vi "根据一字槽的缺口计算旋转矩形找边-计算一字槽角度.vi"(9 "存储缺口位置 out":cluster{"X":sgl, "Y":sgl}[](array[cluster]), 11 "Img输入":T1) -> (0 "一字槽角度线":T2, 1 "角度差异":dbl[](array[numeric]), 2 "一字槽角度":dbl, 3 "Img out":T1, 4 "一字槽宽度":dbl)   [LabVIEW 2014]
uses:
  <vilib>/vision/Measure.llb/Edge Options.ctl
  <vilib>/vision/Measure.llb/Edge Polarity.ctl
  <vilib>/vision/Image Controls.llb/IMAQ Image.ctl
  <vilib>/vision/NI_Vision_Development_Module.lvlib
panel:
  out "Angle2":dbl
  out "Angle1":dbl
  out "角度 2":dbl
  out "角度":dbl
  out "缺口连线角度":dbl
  out "?":dbl[](array[numeric])
  out "槽边与缺口连线差异":dbl
  out "两槽边角度差异":dbl
  in  "Options2":T5={"Search Direction"=1, "Edge Options"={"Edge Polarity"=1, "Kernel Size"=9, "Width"=5, "Minimum Edge Strength"=15.0, "Interpolation Type"=enum."Bilinear Fixed", "Data Processing Method"=enum."Average"}, "Show Search Area"=TRUE, "Show Search Lines"=FALSE, "Show Edges Found"=FALSE, "Show Result"=TRUE, "Search Area Color"=65280, "Search Lines Color"=255, "Edge Locations Color"=16776960, "Result Color"=16711680, "Overlay Group Name"=""} {"Edge Options"."Edge Polarity" items=["All Edges", "Rising Edges", "Falling Edges"]; "Edge Options"."Minimum Edge Strength" format="%.2f"; "Edge Options"."Width" step=2; "Edge Options"."Kernel Size" step=2; "Search Direction" items=["Left to Right", "Right to Left", "Top to Bottom", "Bottom to Top"]}
  in  "Options输入":T5={"Search Direction"=0, "Edge Options"={"Edge Polarity"=1, "Kernel Size"=9, "Width"=3, "Minimum Edge Strength"=15.0, "Interpolation Type"=enum."Bilinear Fixed", "Data Processing Method"=enum."Average"}, "Show Search Area"=TRUE, "Show Search Lines"=FALSE, "Show Edges Found"=FALSE, "Show Result"=TRUE, "Search Area Color"=65280, "Search Lines Color"=255, "Edge Locations Color"=16776960, "Result Color"=16711680, "Overlay Group Name"=""} {"Edge Options"."Edge Polarity" items=["All Edges", "Rising Edges", "Falling Edges"]; "Edge Options"."Minimum Edge Strength" format="%.2f"; "Edge Options"."Width" step=2; "Edge Options"."Kernel Size" step=2; "Search Direction" items=["Left to Right", "Right to Left", "Top to Bottom", "Bottom to Top"]}
  out "两缺口连线角度":dbl
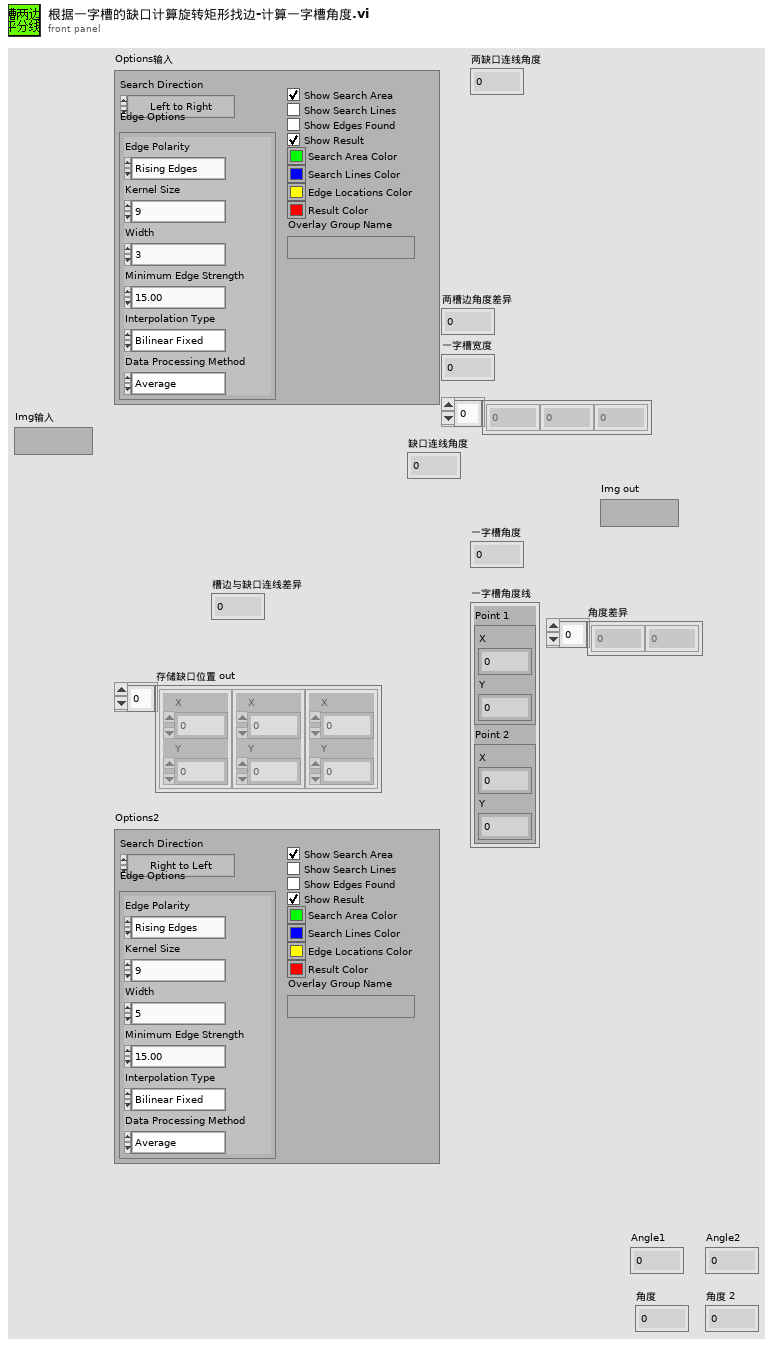
[diagram p1: front panel]
types:
  T1 = typedef "IMAQ Image.ctl" = refnum<image>
  T2 = cluster{"Point 1":cluster{"X":sgl, "Y":sgl}, "Point 2":cluster{"X":sgl, "Y":sgl}}
  T3 = typedef "Edge Options.ctl" = cluster{"Edge Polarity":T4, "Kernel Size":u32, "Width":u32, "Minimum Edge Strength":sgl, "Interpolation Type":enum32{"Zero Order", "Bilinear", "Quadratic", "Cubic", "Bilinear Fixed"}, "Data Processing Method":enum32{"Average", "Median"}}
  T4 = typedef "Edge Polarity.ctl" = u32
  T5 = cluster{"Search Direction":u32, "Edge Options":T3, "Show Search Area":bool, "Show Search Lines":bool, "Show Edges Found":bool, "Show Result":bool, "Search Area Color":u32, "Search Lines Color":u32, "Edge Locations Color":u32, "Result Color":u32, "Overlay Group Name":string}
  T6 = cluster{"Center (Pixels)":cluster{"X":sgl, "Y":sgl}, "Center (Pixels)":cluster{"X":sgl, "Y":sgl}}
  T7 = typedef "ROI Descriptor" = cluster{"Global Rectangle":i32[], "Contours":cluster{"ID":enum32{"External", "Internal"}, "Type":u32, "Coordinates":i32[]}[]}
  T8 = cluster{"Point1 (Pixels)":cluster{"X":sgl, "Y":sgl}, "Point2 (Pixels)":cluster{"X":sgl, "Y":sgl}, "Point1 (Real-World)":cluster{"X":sgl, "Y":sgl}, "Point2 (Real-World)":cluster{"X":sgl, "Y":sgl}, "Angle (Pixel)":dbl, "Angle (Real-World)":dbl, "Score":dbl, "Straightness":dbl, "Average SNR (db)":dbl, "Calibration Valid":bool}[]
  T9 = cluster{"Point1 (Pixels)":cluster{"X":sgl, "Y":sgl}, "Point2 (Pixels)":cluster{"X":sgl, "Y":sgl}, "Point1 (Real-World)":cluster{"X":sgl, "Y":sgl}, "Point2 (Real-World)":cluster{"X":sgl, "Y":sgl}, "Angle (Pixel)":dbl, "Angle (Real-World)":dbl, "Score":dbl, "Straightness":dbl, "Average SNR (db)":dbl, "Calibration Valid":bool}
  T10 = cluster{"Point1 (Pixels)":cluster{"X":sgl, "Y":sgl}, "Point2 (Pixels)":cluster{"X":sgl, "Y":sgl}}
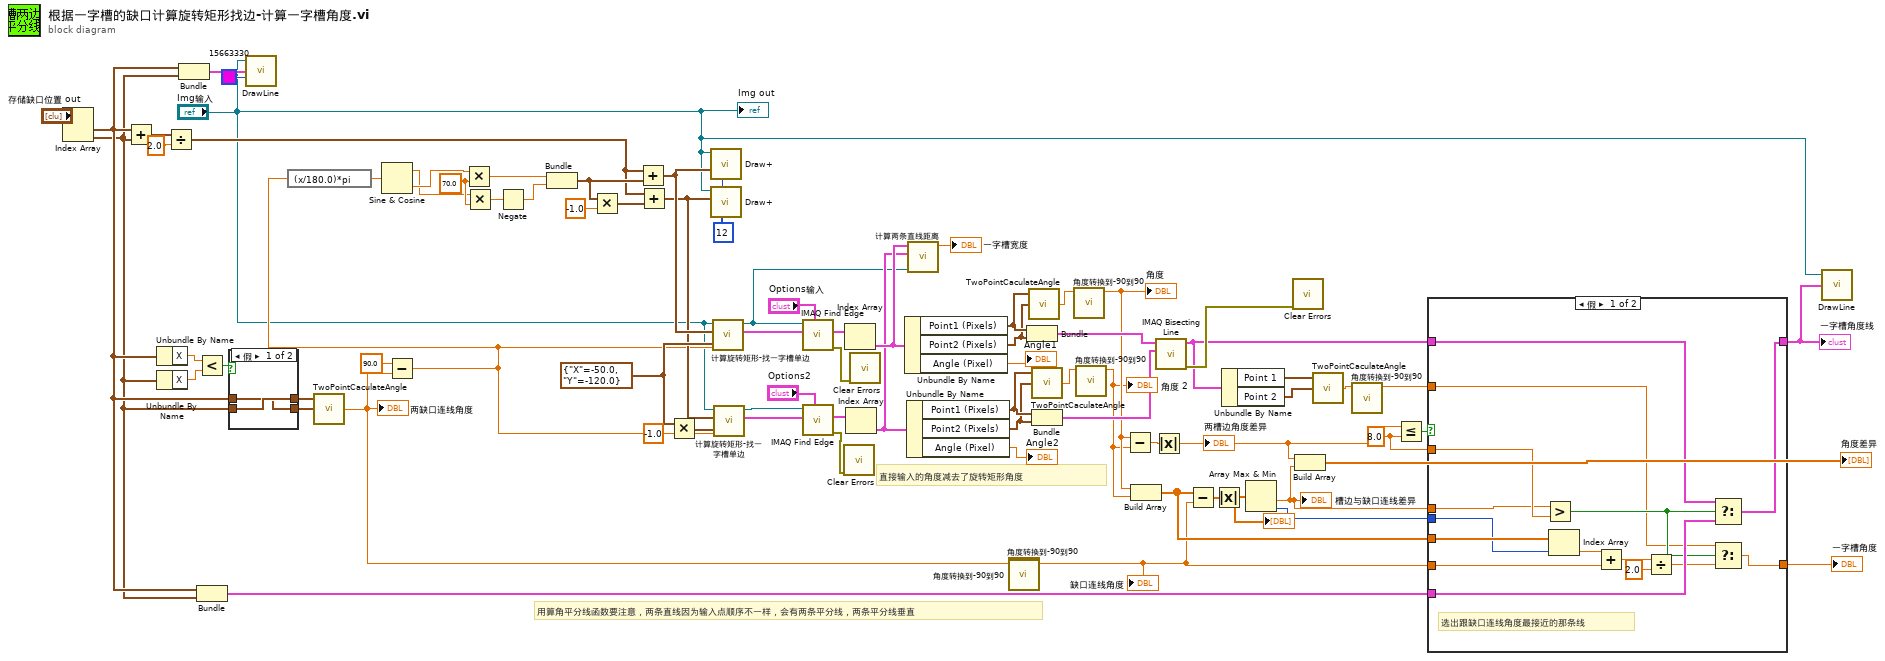
[diagram p0: block diagram]
diagram:
  w29 = 8.0 ("y")
  w45 = 12 ("Width")
  w56 = 70.0 ("y")
  w43 = cluster{"X":dbl, "Y":dbl} {"X"=-50.0, "Y"=-120.0} ("y")
  # "直接输入的角度减去了旋转矩形角度"
  # "用算角平分线函数要注意，两条直线因为输入点顺序不一样，会有两条平分线，两条平分线垂直"
  n1 = Index Array(array="存储缺口位置 out") -> (element #1=w20:cluster{"X":sgl, "Y":sgl}, element #2=w19:cluster{"X":sgl, "Y":sgl})  [unwired: 2 in]
  n2 = Add(x=w20, y=w19) -> (x+y=w63:cluster{"X":sgl, "Y":sgl})
  n3 = Unbundle By Name(w20) -> ("X"=w65:sgl)
  n4 = Unbundle By Name(w19) -> ("X"=w66:sgl)
  n5 = Divide(x=w63, y=2.0) -> (x/y=w50:cluster{"X":dbl, "Y":dbl})
  n6 = Bundle("Center (Pixels)"=w20, "Center (Pixels)"=w19) -> (w49:T6)  [unwired: 1 in]
  n7 = Less?(x=w65, y=w66) -> (x < y?=w67:bool)
  n8 = Bundle("Center (Pixels)"=w20, "Center (Pixels)"=w19) -> (w18:T6)  [unwired: 1 in]
  n9 = case shown="假" w67 {
    tunnel: w20 -> [w79 w82]
    tunnel: w19 -> [w80 w81]
    tunnel: [w80 w82] -> w68
    tunnel: [w79 w81] -> w69
    frame False {
    }
    frame True {
    }
  }
  n10 = call "DrawLine.vi"("Color"=u32 15663330, "Edge Points"=w49, "img in"="Img输入") -> ()  [unwired: 1 out]
  n11 = call "TwoPointCaculateAngle.vi"("Point2"=w69, "Point1"=w68) -> ("角度"=w11:dbl)  [unwired: 1 in]
  "两缺口连线角度" <- w11
  n12 = Subtract(x=90.0, y=w11) -> (x-y=w38:dbl)
  n13 = expression code="(x/180.0)*pi" ("degrees to radians")(w38) -> (w42:dbl)
  n14 = Sine & Cosine(0:w42) -> (1:w47:dbl, 2:w48:dbl)
  n15 = Multiply(x=w48, y=w56) -> (x*y=w57:dbl)
  n16 = Multiply(x=w47, y=w56) -> (x*y=w55:dbl)
  n17 = Negate(x=w55) -> (-x=w54:dbl)
  n18 = Bundle(w57, w54) -> (w53:cluster{dbl, dbl})  [unwired: 1 in]
  n19 = Multiply(x=w53, y=-1.0) -> (x*y=w51:cluster{dbl, dbl})
  n20 = Add(x=w50, y=w53) -> (x+y=w46:cluster{dbl, dbl})
  n21 = Add(x=w50, y=w51) -> (x+y=w39:cluster{dbl, dbl})
  n22 = Multiply(x=w43, y=-1.0) -> (x*y=w40:cluster{"X":dbl, "Y":dbl})
  n23 = call "Draw+.vi"("Width"=w45, "input cluster"=w46, "Image In"="Img输入") -> ()  [unwired: 3 in, 1 out]
  n24 = call "Draw+.vi"("Width"=w45, "input cluster"=w39, "Image In"="Img输入") -> ()  [unwired: 3 in, 1 out]
  n25 = call "计算旋转矩形-找一字槽单边.vi"("矩形"=w43, "旋转角度"=w38, "矩形中心"=w46, "Img输入"="Img输入") -> ("ROI Descriptor"=w37:T7, "Image Out"=w12:T1)  [unwired: 6 in]
  n26 = call "计算旋转矩形-找一字槽单边.vi"("矩形"=w40, "旋转角度"=w38, "矩形中心"=w39, "Img输入"="Img输入") -> ("ROI Descriptor"=w36:T7, "Image Out"=w35:T1)  [unwired: 6 in]
  n27 = call "IMAQ Find Edge"("Options"="Options输入", "ROI Descriptor"=w37, "Image"=w12) -> ("error out"=w17:errorcluster, "Straight Edges"=w72:T8)  [unwired: 5 in, 2 out]
  n28 = call "IMAQ Find Edge"("Options"="Options2", "ROI Descriptor"=w36, "Image"=w35) -> ("error out"=w16:errorcluster, "Straight Edges"=w73:T8)  [unwired: 5 in, 2 out]
  n29 = call <vilib>:"Clear Errors.vi"("error in (no error)"=w16) -> ()  [unwired: 5 in, 2 out]
  n30 = Index Array(array=w72) -> (element=w60:T9)  [unwired: 1 in]
  n31 = Index Array(array=w73) -> (element=w59:T9)  [unwired: 1 in]
  n32 = call <vilib>:"Clear Errors.vi"("error in (no error)"=w17) -> ()  [unwired: 5 in, 2 out]
  n33 = Unbundle By Name(w60) -> ("Point1 (Pixels)"=w10:cluster{"X":sgl, "Y":sgl}, "Point2 (Pixels)"=w9:cluster{"X":sgl, "Y":sgl}, "Angle (Pixel)"=→"Angle1":dbl)
  n34 = Unbundle By Name(w59) -> ("Point1 (Pixels)"=w8:cluster{"X":sgl, "Y":sgl}, "Point2 (Pixels)"=w7:cluster{"X":sgl, "Y":sgl}, "Angle (Pixel)"=→"Angle2":dbl)
  n35 = call "计算两条直线距离.vi"("Img in"=w12, "Straight Edge (下直线)"=w59, "Straight Edge (上直线)"=w60) -> ("Distance"=→"一字槽宽度":dbl)  [unwired: 8 in]
  n36 = call "角度转换到-90到90.vi"() -> ()  [unwired: 11 in, 1 out]
  n37 = call "角度转换到-90到90.vi"("数值输入"=w11) -> ("数值输出"=w25:dbl)  [unwired: 10 in]
  "缺口连线角度" <- w25
  n38 = Bundle("Point1 (Pixels)"=w10, "Point2 (Pixels)"=w9) -> (w62:T10)  [unwired: 1 in]
  n39 = call "TwoPointCaculateAngle.vi"("Point2"=w9, "Point1"=w10) -> ("角度"=w6:dbl)  [unwired: 1 in]
  n40 = call "TwoPointCaculateAngle.vi"("Point2"=w7, "Point1"=w8) -> ("角度"=w4:dbl)  [unwired: 1 in]
  n41 = Bundle("Point1 (Pixels)"=w8, "Point2 (Pixels)"=w7) -> (w74:T10)  [unwired: 1 in]
  n42 = call "角度转换到-90到90.vi"("数值输入"=w6) -> ("数值输出"=w5:dbl)  [unwired: 10 in]
  "角度" <- w5
  n43 = call "角度转换到-90到90.vi"("数值输入"=w4) -> ("数值输出"=w3:dbl)  [unwired: 10 in]
  "角度 2" <- w3
  n44 = Subtract(x=w5, y=w3) -> (x-y=w61:dbl)
  n45 = Build Array(w5, w3) -> (w26:dbl[])
  n46 = Absolute Value(x=w61) -> (abs(x)=w15:dbl)
  "两槽边角度差异" <- w15
  n47 = call "IMAQ Bisecting Line"("Line 2"=w74, "Line 1"=w62) -> ("error out"=w77:errorcluster, "Bisecting Line"=w23:T2)  [unwired: 8 in]
  n48 = Subtract(x=w26, y=w25) -> (x-y=w27:dbl[])
  n49 = Absolute Value(x=w27) -> (abs(x)=w28:dbl[])
  "?" <- w28
  n50 = Unbundle By Name(w23) -> ("Point 1"=w75:cluster{"X":sgl, "Y":sgl}, "Point 2"=w76:cluster{"X":sgl, "Y":sgl})
  n51 = Array Max & Min(array=w28) -> (min value=w14:dbl, min index (indices)=w24:i32)  [unwired: 2 out]
  "槽边与缺口连线差异" <- w14
  n52 = call <vilib>:"Clear Errors.vi"("error in (no error)"=w77) -> ()  [unwired: 5 in, 2 out]
  n53 = Build Array(w15, w14) -> (→"角度差异":dbl[])
  n54 = call "TwoPointCaculateAngle.vi"("Point2"=w76, "Point1"=w75) -> ("角度"=w34:dbl)  [unwired: 1 in]
  n55 = call "角度转换到-90到90.vi"("数值输入"=w34) -> ("数值输出"=w31:dbl)  [unwired: 10 in]
  n56 = Less Or Equal?(x=w15, y=w29) -> (x <= y?=w32:bool)
  n57 = case shown="假" w32 {
    tunnel: w31 -> [w85 w99]
    tunnel: [w83 w99] -> w30
    tunnel: w25 -> [w95 _]
    tunnel: w26 -> [w97 _]
    tunnel: w29 -> [w92 _]
    tunnel: w14 -> [w91 _]
    tunnel: w24 -> [w90 _]
    tunnel: w23 -> [w88 w98]
    tunnel: [w89 w98] -> w21
    tunnel: w18 -> [w87 _]
    frame False {
      # "选出跟缺口连线角度最接近的那条线"
      n58 = Greater?(x=w91, y=w92) -> (0:w86:bool)
      n59 = Index Array(array=w97, index=w90) -> (element=w96:dbl)
      n60 = Add(x=w96, y=w95) -> (x+y=w94:dbl)
      n61 = Divide(x=w94, y=2.0) -> (x/y=w84:dbl)
      n62 = Select(t=w88, s=w86, f=w87) -> (s? t:f=w89:T6)
      n63 = Select(t=w85, s=w86, f=w84) -> (s? t:f=w83:dbl)
    }
    frame True {
    }
  }
  "一字槽角度线" <- w21
  "一字槽角度" <- w30
  n64 = call "DrawLine.vi"("Edge Points"=w21, "img in"="Img输入") -> ()  [unwired: 1 in, 1 out]
  "Img out" <- "Img输入"
